vi "Reply.vi"(7 "Sender":refnum<class "Sender.lvclass">, 9 "Is Priority":bool, 10 "Msg":refnum<class "Msg.lvclass">, 11 "jettl Actor in":refnum<class "jettl Actor.lvclass">) -> (3 "jettl Actor out":refnum<class "jettl Actor.lvclass">)   [LabVIEW 2021, in "jettl.lvlib" / "Temporary Actor.lvlib" / "jettl Actor.lvclass"]
uses:
  jettl Actor.lvclass
  Sender/Sender/Sender.lvclass
  Msg/Msg.lvclass
  jettl Actor.lvclass/jettl Actor.ctl
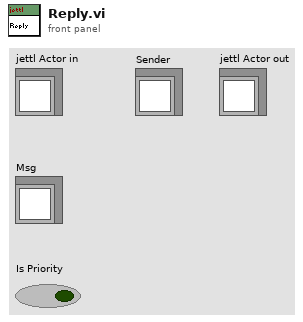
[diagram p1: front panel]
types:
  T1 = typedef "jettl.lvlib/Relation.ctl" = enum16{"Self", "Creator", "Created"}
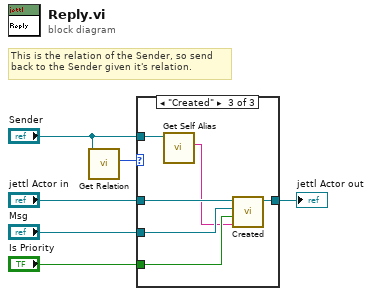
[diagram p0: block diagram]
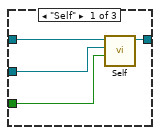
[diagram p2: hidden frame]
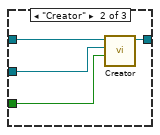
[diagram p3: hidden frame]
diagram:
  # "This is the relation of the Sender, so send back to the Sender given it's relation."
  n1 = call-dynamic "Get Relation.vi"("Sender in"="Sender") -> ("Relation"=w6:T1)  [unwired: 10 in]
  n2 = case shown="\"Created\"" w6 {
    tunnel: [w9 w13 w19] -> w5
    tunnel: "jettl Actor in" -> [w10 w14 w20]
    tunnel: "Msg" -> [w8 w12 w18]
    tunnel: "Is Priority" -> [w7 w11 w17]
    tunnel: "Sender" -> [_ _ w16]
    frame "Self" {
      n3 = call-dynamic "Self.vi"("Is Priority"=w7, "Msg"=w8, "jettl Actor in"=w10) -> ("jettl Actor out"=w9:refnum<class "jettl Actor.lvclass">)  [unwired: 8 in]
    }
    frame "Creator" {
      n4 = call-dynamic "Creator.vi"("Is Priority"=w11, "Msg"=w12, "jettl Actor in"=w14) -> ("jettl Actor out"=w13:refnum<class "jettl Actor.lvclass">)  [unwired: 8 in]
    }
    frame "Created" {
      n5 = call-dynamic "Get Self Alias.vi"("Sender in"=w16) -> ("Self Alias"=w15:string)  [unwired: 10 in]
      n6 = call-dynamic "Created.vi"("Created Alias"=w15, "Is Priority"=w17, "Msg"=w18, "jettl Actor in"=w20) -> ("jettl Actor out"=w19:refnum<class "jettl Actor.lvclass">)  [unwired: 7 in]
    }
  }
  "jettl Actor out" <- w5
